vi "Get Channel Properties.vi"(7 "TypeName":string, 8 "error in":errorcluster, 11 "JSON":string) -> (0 "error out":errorcluster, 3 "Channel Properties":variant)   [LabVIEW 2026, in "NIDMM Deployment Hooks.lvlib"]
uses:
  NIDMM Deployment Hooks.lvlib
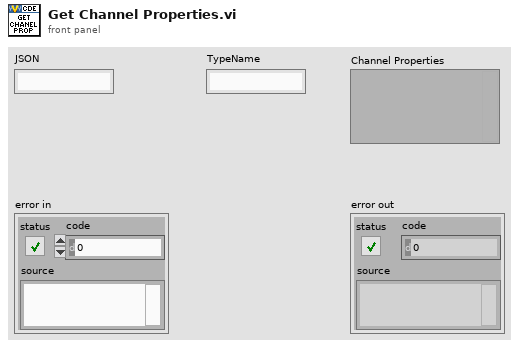
[diagram p1: front panel]
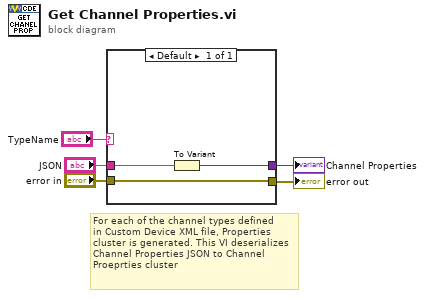
[diagram p0: block diagram]
diagram:
  # "For each of the channel types defined\nin Custom Device XML file, Properties\ncluster is generated. This VI deserializes\nChannel Properties JSON to Channel\nProeprties cluster"
  n1 = case shown="Default" "TypeName" {
    tunnel: [w7] -> w3
    tunnel: "error in" -> [w8]
    tunnel: [w8] -> w4
    tunnel: "JSON" -> [w6]
    frame Default {
      n2 = To Variant(anything=w6) -> (Variant=w7:variant)
    }
  }
  "Channel Properties" <- w3
  "error out" <- w4
